vi "DAQ EOL Create AI Task.vi"(11 "AI Channel In":T1[](array[typedef]) {"input terminal configuration" items=["default"=-1, "RSE"=10083, "NRSE"=10078, "Differential"=10106, "Pseudodifferential"=12529]; "units" items=["Amps"=10342, "Volts"=10348, "From Custom Scale"=10065]}) -> (0 "Error Out":errorcluster, 3 "Analog Input Task":refnum<k21>)   [LabVIEW 2018]
uses:
  02.Type Def's/AIO Channel Configuration Control.ctl
  02.Type Def's/Scalling Configuration Control.ctl
  <vilib>/DAQmx/create/scale.llb/DAQmx Create Scale (Linear).vi
  <vilib>/DAQmx/create/channels.llb/DAQmx Create Channel (AI-Voltage-Basic).vi
  <vilib>/DAQmx/create/channels.llb/DAQmx Create Channel (AI-Temperature-Thermocouple).vi
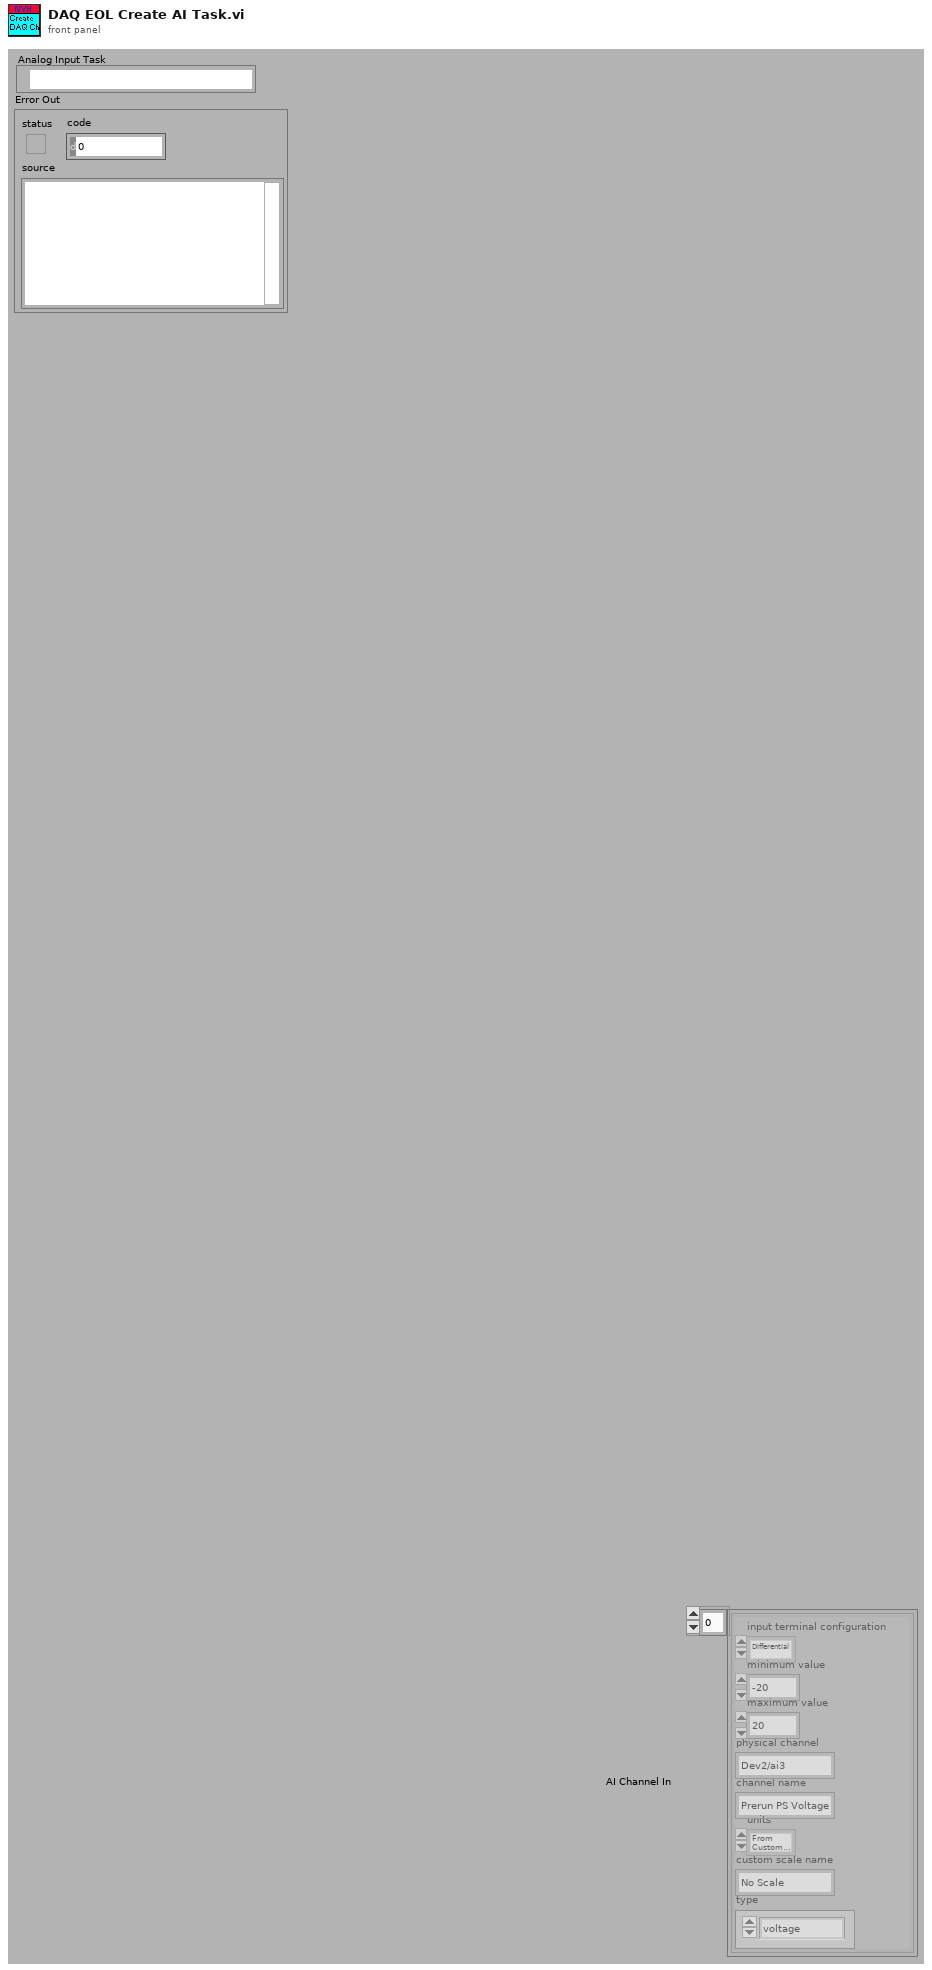
[diagram p1: front panel]
types:
  T1 = typedef "AIO Channel Configuration Control.ctl" = cluster{"input terminal configuration":i32, "minimum value":dbl, "maximum value":dbl, "physical channel":string, "channel name":string, "units":i32, "custom scale name":string, "type":enum16{"voltage", "thermocouple", "Amps"}}
  T2 = typedef "Scalling Configuration Control.ctl" = cluster{"name":string, "slope":dbl}
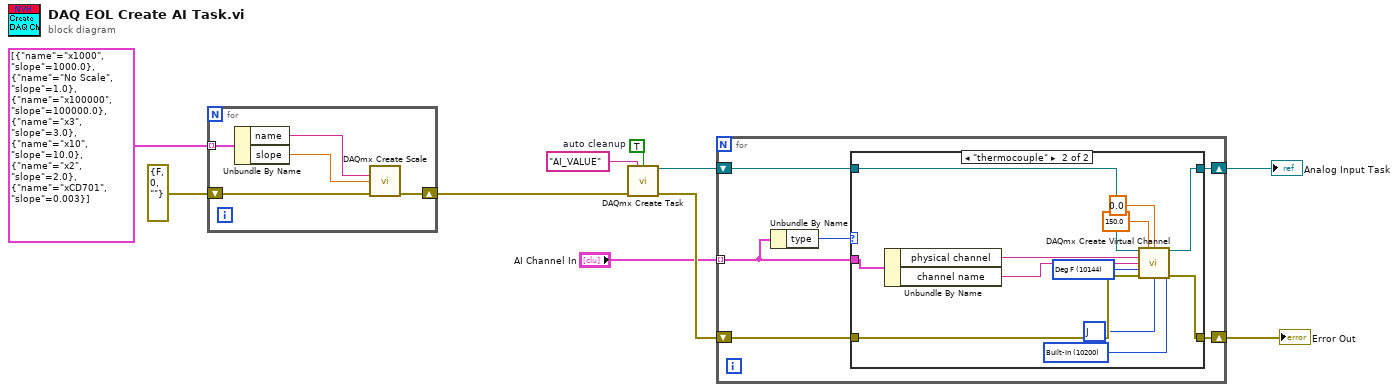
[diagram p0: block diagram]
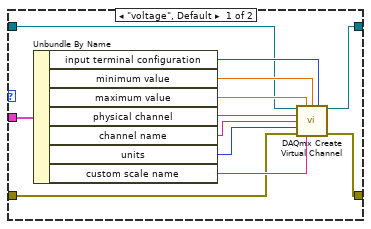
[diagram p2: hidden frame]
diagram:
  w10 = TRUE  # auto cleanup
  n1 = for {
    shift-right: [w15] -> w9
    shift-left: errorcluster {"status"=FALSE, "code"=0, "source"=""} ("error out") -> [w14]
    tunnel: T2[] [{"name"="x1000", "slope"=1000.0}, {"name"="No Scale", "slope"=1.0}, {"name"="x100000", "slope"=100000.0}, {"name"="x3", "slope"=3.0}, {"name"="x10", "slope"=10.0}, {"name"="x2", "slope"=2.0}, {"name"="xCD701", "slope"=0.003}] -> [w13] mode=indexing
    n2 = Unbundle By Name(w13) -> ("name"=w12:string, "slope"=w11:dbl)
    n3 = call-poly <vilib>:"DAQmx Create Scale.vi"("name"=w12, "slope"=w11, "error in"=w14) -> ("error out"=w15:errorcluster)  [unwired: 3 in, 9 out]
  }
  n4 = call <vilib>:"DAQmx Create Task.vi"("new task name"="AI_VALUE", "auto cleanup"=w10, "error in"=w9) -> ("task out"=w8:refnum<k21>, "error out"=w7:errorcluster)  [unwired: 2 in, 9 out]
  n5 = for {
    tunnel: "AI Channel In" -> [w17] mode=indexing
    shift-right: [w20] -> w4
    shift-left: w8 -> [w21]
    shift-right: [w18] -> w3
    shift-left: w7 -> [w19]
    n6 = Unbundle By Name(w17) -> ("type"=w16:enum16{"voltage", "thermocouple", "Amps"})
    n7 = case shown="\"thermocouple\"" w16 {
      tunnel: w17 -> [w33 w45]
      tunnel: w21 -> [w25 w42]
      tunnel: [w24 w41] -> w20
      tunnel: w19 -> [w23 w40]
      tunnel: [w22 w39] -> w18
      frame "voltage", Default {
        n8 = Unbundle By Name(w33) -> ("input terminal configuration"=w32:i32, "minimum value"=w31:dbl, "maximum value"=w30:dbl, "physical channel"=w29:string, "channel name"=w28:string, "units"=w27:i32, "custom scale name"=w26:string)
        n9 = call-poly <vilib>:"DAQmx Create Virtual Channel.vi"("task in"=w25, "maximum value"=w30, "minimum value"=w31, "input terminal configuration"=w32, "physical channels"=w29, "name to assign"=w28, "units"=w27, "error in"=w23, "custom scale name"=w26) -> ("task out"=w24:refnum<k21>, "error out"=w22:errorcluster)  [unwired: 5 out]
      }
      frame "thermocouple" {
        w34 = 10144 items=["Deg C"=10143, "Deg F"=10144, "Kelvins"=10325, "Deg R"=10145, "From Custom Scale"=10065] ("units")
        w37 = 10200 items=["Built-In"=10200, "Constant Value"=10116, "Channel"=10113] ("cjc source")
        w38 = 10072 items=["J"=10072, "K"=10073, "N"=10077, "R"=10082, "S"=10085, "T"=10086, "B"=10047, "E"=10055] ("thermocouple type")
        n10 = Unbundle By Name(w45) -> ("physical channel"=w44:string, "channel name"=w43:string)
        n11 = call-poly <vilib>:"DAQmx Create Virtual Channel.vi"("task in"=w42, "maximum value"=150.0, "minimum value"=0.0, "physical channels"=w44, "cjc source"=w37, "name to assign"=w43, "units"=w34, "error in"=w40, "thermocouple type"=w38) -> ("task out"=w41:refnum<k21>, "error out"=w39:errorcluster)  [unwired: 4 in, 1 out]
      }
    }
  }
  "Analog Input Task" <- w4
  "Error Out" <- w3
